vi "Close.vi"(8 "error in":errorcluster, 11 "DB-MySQL in":refnum<class "DB-MySQL.lvclass">=refnum) -> (0 "error out":errorcluster, 3 "DB-MySQL out":refnum<class "DB-MySQL.lvclass">)   [LabVIEW 2022 SP3, in "hse-db-mysql.lvlib" / "DB-MySQL.lvclass"]
doc: "____\nHAMPEL SOFTWARE ENGINEERING v1.4.0 (2023-12-19 09:52)"
uses:
  DB-MySQL.lvclass
  DB-MySQL.lvclass/DB-MySQL.ctl
  <vilib>/Hampel Software Engineering/MySQLNetCom/MySQLNetCom.lvlib
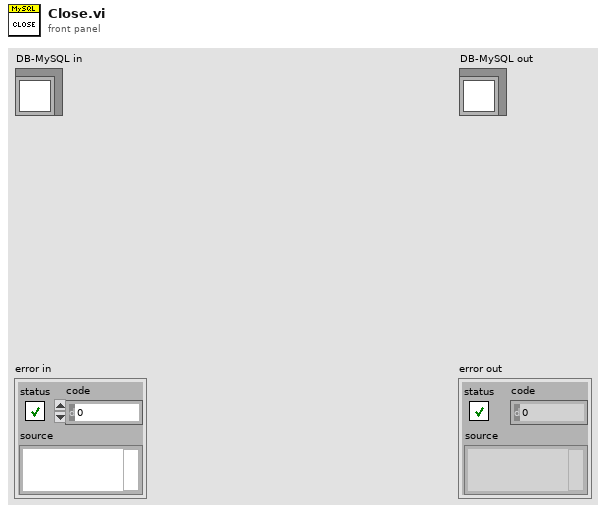
[diagram p1: front panel]
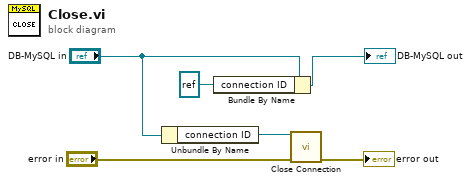
[diagram p0: block diagram]
diagram:
  n1 = Unbundle By Name("DB-MySQL in") -> ("connection ID"=w2:refnum<k5>)
  n2 = Bundle By Name(cluster="DB-MySQL in", "connection ID"=refnum<k5> refnum ("connection ID out")) -> (→"DB-MySQL out":refnum<class "DB-MySQL.lvclass">)
  n3 = call <vilib>:"Close Connection.vi"("connection ID"=w2, "error in (no error)"="error in") -> ("error out"=→"error out":errorcluster)  [unwired: 13 in]
